vi "Untitled 2.vi"() -> ()   [LabVIEW 2015, in "DBToolkit.lvlib"]
uses:
  DBToolkit.lvlib
  <vilib>/Utility/miscctls.llb/LVDateTimeRec.ctl
  <vilib>/drjdpowell/SQLite Library/SQL Statement/SQL Statement.lvclass/SQL Statement.ctl
  <vilib>/drjdpowell/SQLite Library/SQL Statement/Bind Timestamp (Text).vi
  <vilib>/drjdpowell/SQLite Library/SQL Statement/Bind Text.vi
  <vilib>/drjdpowell/SQLite Library/SQL Statement/Error Message.vi
  <vilib>/drjdpowell/SQLite Library/SQL Statement/Column Timestamp.vi
  <vilib>/drjdpowell/SQLite Library/SQL Statement/Column String.vi
  <vilib>/drjdpowell/SQLite Library/SQL Statement/Column Path.vi
  <vilib>/drjdpowell/SQLite Library/SQL Connection/Connection.lvclass
  <vilib>/drjdpowell/SQLite Library/SQL Statement/SQL Statement.lvclass
  FileHandler/FileHandler.lvlib
panel:
  in  "time stamp":timestamp
  out "SQLite Time String":string
  out "Array":timestamp[](array[timestamp])
  out "x-y":timestamp
  in  "Days":i32
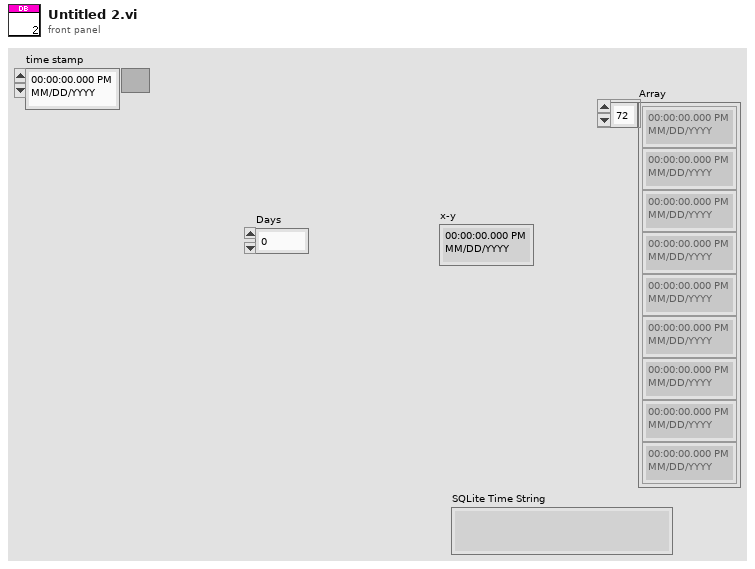
[diagram p1: front panel]
types:
  T1 = typedef "LVDateTimeRec.ctl" = cluster{"fractional second":dbl, "second":i32, "minute":i32, "hour":i32, "day of month":i32, "month":i32, "year":i32, "day of week":i32, "day of year":i32, "DST":i32}
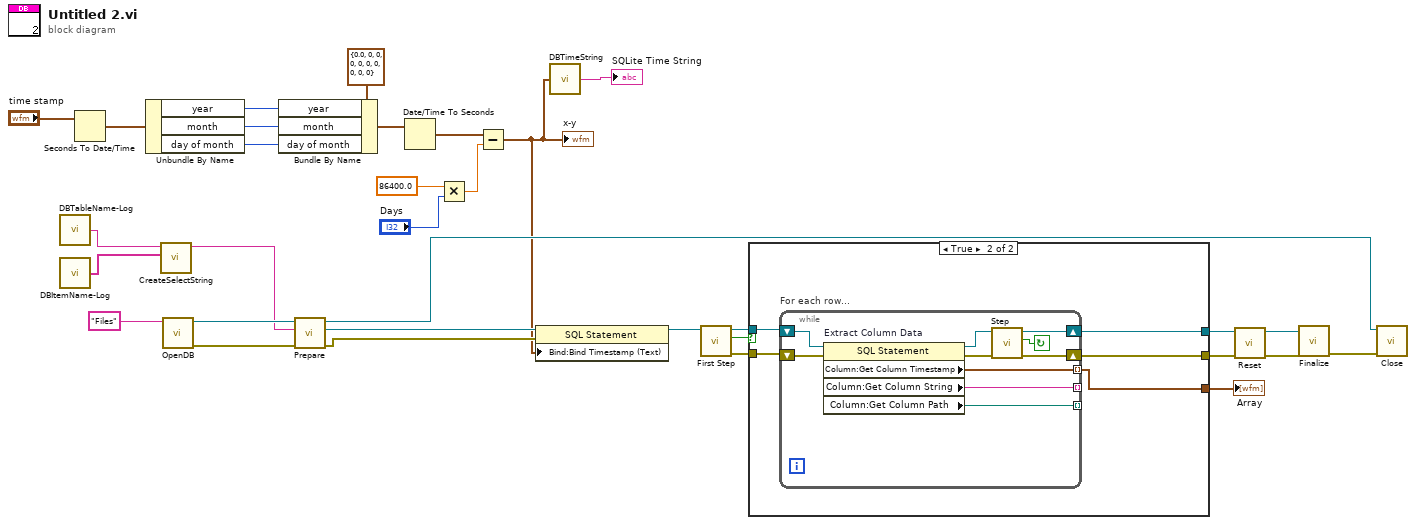
[diagram p0: block diagram]
diagram:
  n1 = call "DBTableName-Log.vi"() -> ("DB Table Name"=w1:string)  [unwired: 5 in]
  n2 = call "DBItemName-Log.vi"() -> ("Items"=w2:string[])  [unwired: 5 in]
  n3 = Seconds To Date/Time(time stamp (now)="time stamp") -> (date time rec=w31:T1)  [unwired: 1 in]
  n4 = Unbundle By Name(w31) -> ("year"=w30:i32, "month"=w29:i32, "day of month"=w28:i32)
  n5 = call "CreateSelectString.vi"("Items"=w2, "Table Name"=w1) -> ("Create Select String (by Time)"=w3:string)  [unwired: 9 in]
  n6 = call "OpenDB.vi"("DB File Name"="Files") -> ("error out"=w20:errorcluster, "SQLite Connection out"=w21:refnum<class "Connection.lvclass">)  [unwired: 9 in]
  n7 = Bundle By Name(cluster=T1 {"fractional second"=0.0, "second"=0, "minute"=0, "hour"=0, "day of month"=0, "month"=0, "year"=0, "day of week"=0, "day of year"=0, "DST"=0} ("date time rec"), "year"=w30, "month"=w29, "day of month"=w28) -> (w27:T1)
  n8 = call <vilib>:"Prepare.vi"("error in (no error)"=w20, "SQL"=w3, "SQLite Connection in"=w21) -> ("error out"=w8:errorcluster, "SQL Statement out"=w19:refnum<class "SQL Statement.lvclass">, "SQLite Connection out"=w9:refnum<class "Connection.lvclass">)  [unwired: 4 in, 2 out]
  n9 = Date/Time To Seconds(2:w27) -> (0:w26:timestamp)  [unwired: 1 in]
  n10 = Multiply(x=86400.0, y="Days") -> (x*y=w23:dbl)
  n11 = Subtract(x=w26, y=w23) -> (x-y=w4:timestamp)
  "x-y" <- w4
  n12 = property class="SQL Statement"(reference=w19, error in=w8, "Bind:Bind Timestamp (Text)"=w4) -> (reference out=w18:refnum<class "SQL Statement.lvclass">)  [unwired: 1 out]
  n13 = call "DBTimeString.vi"("Time Stamp"=w4) -> ("SQLite Time String"=→"SQLite Time String":string)  [unwired: 4 in]
  n14 = call <vilib>:"First Step.vi"("SQL Statement in"=w18) -> ("error out"=w16:errorcluster, "Row returned"=w15:bool, "SQL Statement out"=w17:refnum<class "SQL Statement.lvclass">)  [unwired: 8 in]
  n15 = case shown="True" w15 {
    tunnel: w17 -> [w33 w39]
    tunnel: w16 -> [w34 w38]
    tunnel: [w34 w37] -> w13
    tunnel: [w33 w36] -> w14
    tunnel: [_ w35] -> w5
    frame False {
    }
    frame True {
      n16 = while "For each row..." {
        shift-right: [w48] -> w36
        shift-left: w39 -> [w45]
        shift-right: [w46] -> w37
        shift-left: w38 -> [w44]
        tunnel: [w42] -> _ mode=indexing
        tunnel: [w41] -> _ mode=indexing
        tunnel: [w40] -> w35 mode=indexing
        stop <- w43 continue-if-true
        n17 = property on="Extract Column Data" class="SQL Statement"(reference=w45, error in=w44) -> (reference out=w49:refnum<class "SQL Statement.lvclass">, error out=w47:errorcluster, "Column:Get Column Timestamp"=w40:timestamp, "Column:Get Column String"=w42:string, "Column:Get Column Path"=w41:path)
        n18 = call <vilib>:"Step.vi"("error in (no error)"=w47, "SQL Statement in"=w49) -> ("error out"=w46:errorcluster, "Row returned"=w43:bool, "SQL Statement out"=w48:refnum<class "SQL Statement.lvclass">)  [unwired: 7 in]
      }
    }
  }
  "Array" <- w5
  n19 = call <vilib>:"Reset.vi"("error in (no error)"=w13, "SQL Statement in"=w14) -> ("error out"=w11:errorcluster, "SQL Statement out"=w12:refnum<class "SQL Statement.lvclass">)  [unwired: 8 in]
  n20 = call <vilib>:"Finalize.vi"("error in (no error)"=w11, "SQL Statement in"=w12) -> ("error out"=w10:errorcluster)  [unwired: 9 in]
  n21 = call-dynamic "Close.vi"("error in (no error)"=w10, "SQLite Connection in"=w9) -> ()  [unwired: 9 in, 1 out]
